vi "dfd_Kaiser Parameters.vi"(6 "fs [Hz]":dbl=1.0 format="%.2f", 8 "error in (no error)":errorcluster, 9 "A stop [dB]":dbl=72.0 format="%.2f", 11 "delta f [Hz]":dbl=0.1 format="%.2f") -> (0 "error out":errorcluster, 1 "beta":dbl format="%.2f", 2 "order for fb":dbl, 3 "order":i32)   [LabVIEW 2017, in "NI_DigFilterLicensed.lvlib"]
uses:
  <vilib>/addons/Digital Filter Design/NI_DigFilterLicensed.lvlib
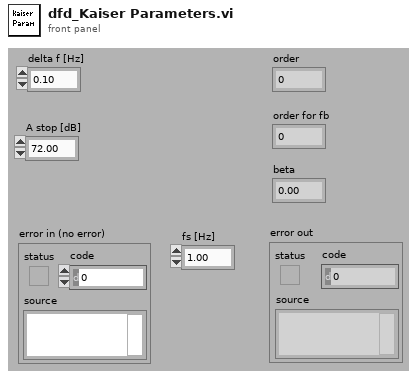
[diagram p1: front panel]
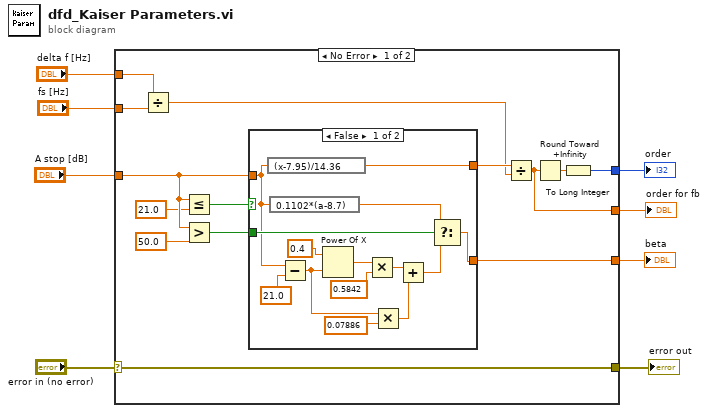
[diagram p0: block diagram]
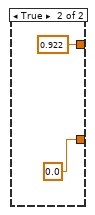
[diagram p2: hidden frame]
diagram:
  n1 = case shown="No Error" "error in (no error)" {
    selector: "error in (no error)" -> [w9 w39]
    tunnel: [w22 _] -> w8
    tunnel: "A stop [dB]" -> [w20 _]
    tunnel: "fs [Hz]" -> [w15 _]
    tunnel: "delta f [Hz]" -> [w14 _]
    tunnel: [w11 _] -> w4
    tunnel: [w10 _] -> w3
    tunnel: [w9 w39] -> w1
    frame No Error {
      n2 = Divide(x=w14, y=w15) -> (x/y=w12:dbl)
      n3 = Less Or Equal?(x=w20, y=21.0) -> (x <= y?=w18:bool)
      n4 = Greater?(x=w20, y=50.0) -> (0:w19:bool)
      n5 = case shown="False" w18 {
        tunnel: [w35 0.0] -> w22
        tunnel: [w36 0.922] -> w13
        tunnel: w19 -> [w34 _]
        tunnel: w20 -> [w32 _]
        frame False {
          n6 = expression code="(x-7.95)/14.36"(w32) -> (w36:dbl)
          n7 = expression code="0.1102*(a-8.7)"(w32) -> (w33:dbl)
          n8 = Subtract(x=w32, y=21.0) -> (x-y=w26:dbl)
          n9 = Power Of X(1:w26, 2:0.4 ("y")) -> (0:w29:dbl)
          n10 = Multiply(x=w29, y=0.5842) -> (x*y=w25:dbl)
          n11 = Multiply(x=w26, y=0.07886) -> (x*y=w24:dbl)
          n12 = Add(x=w25, y=w24) -> (x+y=w23:dbl)
          n13 = Select(t=w33, s=w34, f=w23) -> (s? t:f=w35:dbl)
        }
        frame True {
        }
      }
      n14 = Divide(x=w13, y=w12) -> (x/y=w11:dbl)
      n15 = Round Toward +Infinity(x=w11) -> (ceil(x): smallest int >= x=w21:dbl)
      n16 = To Long Integer(number=w21) -> (32bit integer=w10:i32)
    }
    frame Error {
    }
  }
  "order" <- w3
  "beta" <- w8
  "order for fb" <- w4
  "error out" <- w1
